vi "HSL to Colour.vi"(8 "error in (no error)":errorcluster, 9 "Lightness(%)":dbl format="%#_13g", 10 "Saturation(%)":dbl format="%#_13g", 11 "Hue(°)":dbl format="%#_13g") -> (0 "error out":errorcluster, 3 "Color":u32(colorbox))   [LabVIEW 2018, in "Colour Lab.lvlib"]
uses:
  Colour Lab.lvlib
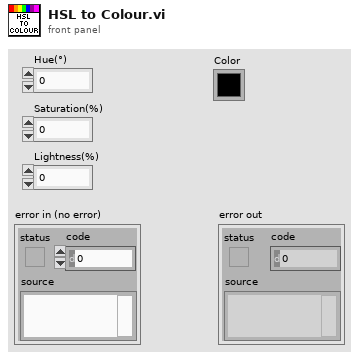
[diagram p1: front panel]
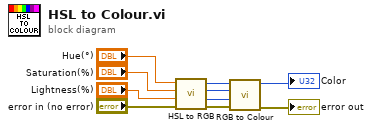
[diagram p0: block diagram]
diagram:
  n1 = call "HSL to RGB.vi"("error in (no error)"="error in (no error)", "Lightness(%)"="Lightness(%)", "Saturation(%)"="Saturation(%)", "Hue(°)"="Hue(°)") -> ("error out"=w10:errorcluster, "Blue"=w9:u8, "Green"=w8:u8, "Red"=w7:u8)  [unwired: 4 in]
  n2 = call "RGB to Colour.vi"("error in (no error)"=w10, "Blue"=w9, "Green"=w8, "Red"=w7) -> ("error out"=→"error out":errorcluster, "Color"=→"Color":u32)  [unwired: 6 in]
